vi "Condition String.vi"(8 "error in (no error)":errorcluster, 9 "input string":string) -> (0 "error out":errorcluster, 1 "result string":string)   [LabVIEW 2024, in "Generic Config Handling.lvlib"]
doc: "Replaces spaces with underscores. Use this to condition key and section names."
uses:
  Generic Config Handling.lvlib
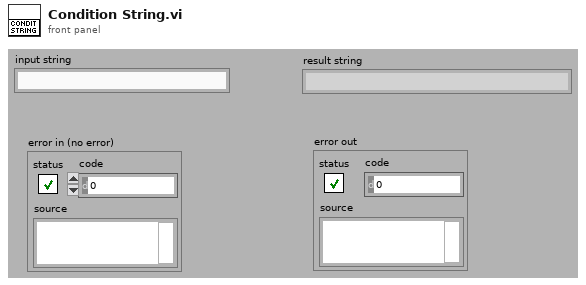
[diagram p1: front panel]
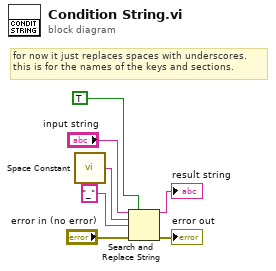
[diagram p0: block diagram]
diagram:
  # "for now it just replaces spaces with underscores.\nthis is for the names of the keys and sections."
  n1 = call <vilib>:"Space Constant.vi"() -> ("String"=w1:string)
  n2 = Search and Replace String(replace all?=TRUE ("replace all? (F)"), input string="input string", search string=w1, replace string="_" ("replace string (\"\")"), error in="error in (no error)") -> (result string=→"result string":string, error out=→"error out":errorcluster)  [unwired: 3 in, 2 out]
